vi "Lookup Module class.vi"() -> (0 "error out":errorcluster, 2 "Enum":T1(c390))   [LabVIEW 2021]
uses:
  <vilib>/Javier Lopez/Configuration File/Json Element/Build_Javier_Lopez_lib_Configuration_Filejson class.lvclass
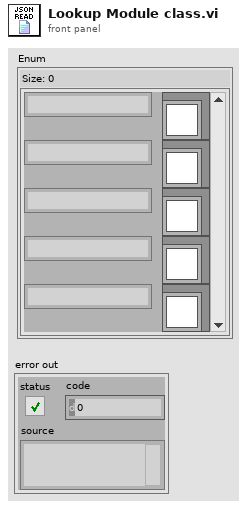
[diagram p1: front panel]
types:
  T1 = map{string, refnum<class "Build_Javier_Lopez_lib_Configuration_Filejson class.lvclass">}
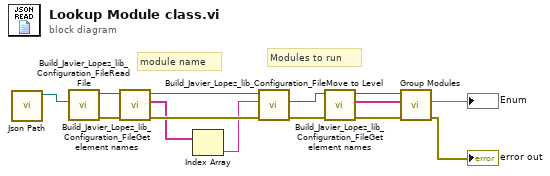
[diagram p0: block diagram]
diagram:
  # "Modules to run"
  # "module name"
  n1 = call "Json Path.vi"() -> ("Path"=w14:path)  [unwired: 11 in]
  n2 = call <vilib>:"Build_Javier_Lopez_lib_Configuration_FileRead File.vi"("Path"=w14) -> ("error out"=w11:errorcluster, "json class out"=w13:refnum<class "Build_Javier_Lopez_lib_Configuration_Filejson class.lvclass">)  [unwired: 9 in]
  n3 = call-dynamic "Build_Javier_Lopez_lib_Configuration_FileGet element names.vi"("error in (no error)"=w11, "json class in"=w13) -> ("error out"=w10:errorcluster, "Item Names"=w9:string[], "json class out"=w12:refnum<class "Build_Javier_Lopez_lib_Configuration_Filejson class.lvclass">)  [unwired: 7 in]
  n4 = Index Array(array=w9) -> (element=w8:string)  [unwired: 1 in]
  n5 = call-dynamic "Build_Javier_Lopez_lib_Configuration_FileMove to Level.vi"("error in (no error)"=w10, "Element"=w8, "json class in"=w12) -> ("error out"=w6:errorcluster, "New json class"=w7:refnum<class "Build_Javier_Lopez_lib_Configuration_Filejson class.lvclass">)  [unwired: 6 in, 1 out]
  n6 = call-dynamic "Build_Javier_Lopez_lib_Configuration_FileGet element names.vi"("error in (no error)"=w6, "json class in"=w7) -> ("error out"=w3:errorcluster, "Item Names"=w2:string[], "json class out"=w4:refnum<class "Build_Javier_Lopez_lib_Configuration_Filejson class.lvclass">)  [unwired: 7 in]
  n7 = call "Group Modules.vi"("error in"=w3, "Item Names"=w2, "json class out"=w4) -> ("error out"=→"error out":errorcluster, "Enum"=→"Enum":T1)  [unwired: 7 in]
